vi "get_data.vi"(8 "error in (no error)":errorcluster, 11 "Experiment in":refnum<class "Experiment.lvclass">) -> (0 "error out":errorcluster, 3 "Experiment out":refnum<class "Experiment.lvclass">)   [LabVIEW 2013, in "Experiment.lvclass"]
uses:
  Experiment.lvclass
  Experiment.lvclass/Experiment.ctl
  Counter/Counter.lvclass
  Camera/Hamamatsu_C9100-13/Hamamatsu_C9100-13.lvclass
  Globals.vi
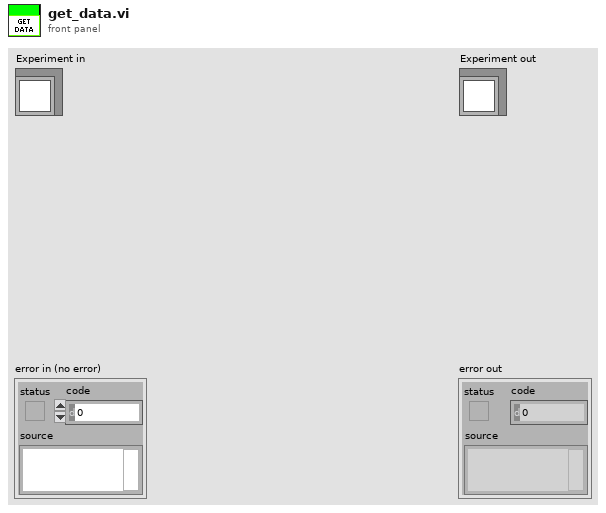
[diagram p1: front panel]
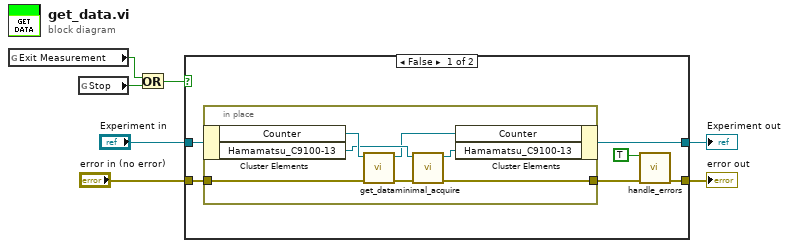
[diagram p0: block diagram]
diagram:
  n1 = global read "Globals.vi" "Exit Measurement"() -> (w3:bool)
  n2 = global read "Globals.vi" "Stop"() -> (w2:bool)
  n3 = Or(x=w3, y=w2) -> (x .or. y?=w1:bool)
  n4 = case shown="False" w1 {
    tunnel: "error in (no error)" -> [w13 w21]
    tunnel: [w11 w21] -> w6
    tunnel: "Experiment in" -> [w10 w22]
    tunnel: [w9 w22] -> w4
    frame False {
      n5 = in-place {
        in-place-border: w13 -> [w20]
        in-place-border: [w14] -> w12
        n6 = in-place-cluster #1(w10) -> ("Counter"=w19:refnum<class "Counter.lvclass">, "Hamamatsu_C9100-13"=w18:refnum<class "Hamamatsu_C9100-13.lvclass">)
        n7 = call-dynamic "get_data.vi"("error in (no error)"=w20, "Counter in"=w19) -> ("error out"=w16:errorcluster, "Counter out"=w17:refnum<class "Counter.lvclass">)  [unwired: 8 in]
        n8 = call-dynamic "minimal_acquire.vi"("error in (no error)"=w16, "Hamamatsu_C9100-13 in"=w18) -> ("error out"=w14:errorcluster, "Hamamatsu_C9100-13 out"=w15:refnum<class "Hamamatsu_C9100-13.lvclass">)  [unwired: 8 in]
        n9 = in-place-cluster #1("Counter"=w17, "Hamamatsu_C9100-13"=w15) -> (w9:refnum<class "Experiment.lvclass">)
      }
      n10 = call "handle_errors.vi"("Exit Operation"=TRUE ("Exit Measurement"), "error in (no error)"=w12) -> ("error out"=w11:errorcluster)  [unwired: 13 in]
    }
    frame True {
    }
  }
  "error out" <- w6
  "Experiment out" <- w4
